vi "SET_ScrollbarPosition.vi"(8 "error in (no error)":errorcluster, 10 "Scrollbar Position":i32, 11 "FakedArray.lvclass in":refnum<class "FakedArray.lvclass">) -> (0 "error out":errorcluster, 3 "FakedArray.lvclass out":refnum<class "FakedArray.lvclass">)   [LabVIEW 2021, in "FakedArray.lvclass"]
uses:
  <resource>/plugins/NIIconEditor/Class/FakedArray/FakedArray.lvclass
  <resource>/plugins/NIIconEditor/Class/FakedArray/FakedArray.lvclass/FakedArray.ctl
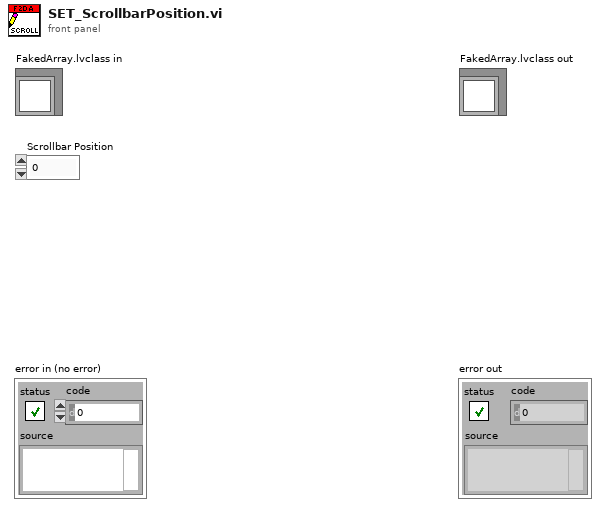
[diagram p1: front panel]
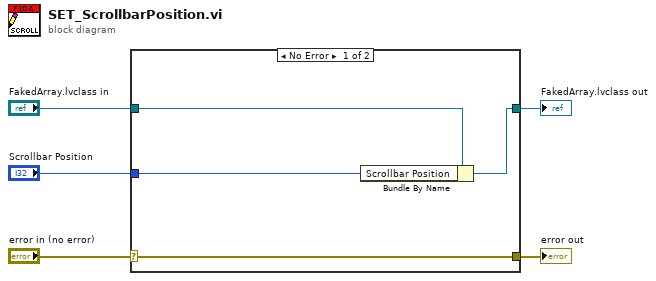
[diagram p0: block diagram]
diagram:
  n1 = case shown="No Error" "error in (no error)" {
    selector: "error in (no error)" -> [w9 w10]
    tunnel: [w9 w10] -> w4
    tunnel: [w7 w11] -> w2
    tunnel: "FakedArray.lvclass in" -> [w8 w11]
    tunnel: "Scrollbar Position" -> [w6 _]
    frame No Error {
      n2 = Bundle By Name(cluster=w8, "Scrollbar Position"=w6) -> (w7:refnum<class "FakedArray.lvclass">)
    }
    frame Error {
    }
  }
  "error out" <- w4
  "FakedArray.lvclass out" <- w2
